vi "Columns.vi"() -> (2 "Columns":T1)   [LabVIEW 2020, in "Test.lvlib" / "Player.lvclass"]
uses:
  Player.lvclass
  Player.lvclass/Player.ctl
  <vilib>/IlluminatedG/IG Conditum Base/Conditum/Columns/Type/Definition.ctl
  <vilib>/IlluminatedG/IG Conditum Base/Conditum/Columns/Type/Type.lvclass
  <vilib>/IlluminatedG/IG Conditum Base/Conditum/Attributes.ctl
  <vilib>/IlluminatedG/IG Conditum Base/Conditum/Conditum.lvlib
  <vilib>/IlluminatedG/IG Conditum Base/Conditum/Columns/String/Definition.ctl
  <vilib>/IlluminatedG/IG Conditum Base/Conditum/Columns/String/String.lvclass
  <vilib>/IlluminatedG/IG Conditum Base/Conditum/Columns/String/String Definition.ctl
  <vilib>/IlluminatedG/IG Conditum Base/Conditum/Columns/Double/Definition.ctl
  <vilib>/IlluminatedG/IG Conditum Base/Conditum/Columns/Double/Double.lvclass
  <vilib>/IlluminatedG/IG Conditum Base/Conditum/Columns/Double/Double Definition.ctl
  <vilib>/IlluminatedG/IG Conditum Base/Conditum/Columns/Boolean/Definition.ctl
  <vilib>/IlluminatedG/IG Conditum Base/Conditum/Columns/Boolean/Boolean.lvclass
  <vilib>/IlluminatedG/IG Conditum Base/Conditum/Columns/Boolean/Boolean Definition.ctl
  C:/Program Files (x86)/National Instruments/LabVIEW 2020/vi.lib/IlluminatedG/IG Conditum Base/Conditum/Columns/Type/Type.lvclass
  C:/Program Files (x86)/National Instruments/LabVIEW 2020/vi.lib/IlluminatedG/IG Conditum Base/Conditum/Columns/String/String.lvclass
  C:/Program Files (x86)/National Instruments/LabVIEW 2020/vi.lib/IlluminatedG/IG Conditum Base/Conditum/Columns/Double/Double.lvclass
  C:/Program Files (x86)/National Instruments/LabVIEW 2020/vi.lib/IlluminatedG/IG Conditum Base/Conditum/Columns/Boolean/Boolean.lvclass
  Columns.ctl
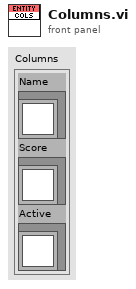
[diagram p1: front panel]
types:
  T1 = typedef "Test.lvlib/Player.lvclass/Columns.ctl" = cluster{"Name":refnum<class "String.lvclass">, "Score":refnum<class "Double.lvclass">, "Active":refnum<class "Boolean.lvclass">}
  T2 = typedef "Conditum.lvlib/Columns.lvlib/Boolean.lvclass/Boolean Definition.ctl" = cluster{"Type":T3, "Attributes":T4, "Boolean":T5}
  T3 = typedef "Conditum.lvlib/Columns.lvlib/Type.lvclass/Definition.ctl" = cluster{"Name":string, "Nullable":bool, "Default NULL":bool}
  T4 = typedef "Conditum.lvlib/Attributes.ctl" = cluster{"Primary Key":bool, "Unique":bool, "Foreign Key":bool, "Auto Increment":bool}
  T5 = typedef "Conditum.lvlib/Columns.lvlib/Boolean.lvclass/Definition.ctl" = cluster{"Default":bool}
  T6 = typedef "Conditum.lvlib/Columns.lvlib/Double.lvclass/Double Definition.ctl" = cluster{"Type":T3, "Attributes":T4, "Double":T7}
  T7 = typedef "Conditum.lvlib/Columns.lvlib/Double.lvclass/Definition.ctl" = cluster{"Default":dbl}
  T8 = typedef "Conditum.lvlib/Columns.lvlib/String.lvclass/String Definition.ctl" = cluster{"Type":T3, "Attributes":T4, "String":T9}
  T9 = typedef "Conditum.lvlib/Columns.lvlib/String.lvclass/Definition.ctl" = cluster{"Default":string, "Length":i32}
  T10 = cluster{"String out":refnum<class "String.lvclass">, "Double out":refnum<class "Double.lvclass">, "Boolean out":refnum<class "Boolean.lvclass">}
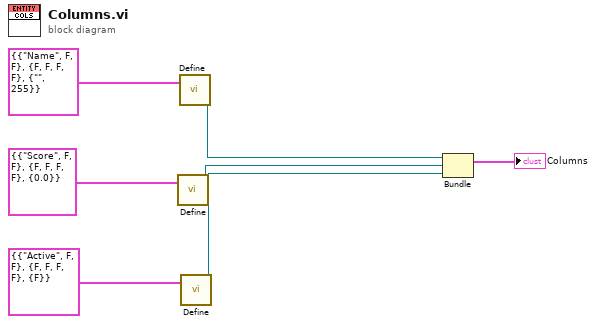
[diagram p0: block diagram]
diagram:
  n1 = call <vilib>:"Define.vi"("Double Definition"=T6 {"Type"={"Name"="Score", "Nullable"=FALSE, "Default NULL"=FALSE}, "Attributes"={"Primary Key"=FALSE, "Unique"=FALSE, "Foreign Key"=FALSE, "Auto Increment"=FALSE}, "Double"={"Default"=0.0}}) -> ("Double out"=w3:refnum<class "Double.lvclass">)  [unwired: 10 in]
  n2 = call <vilib>:"Define.vi"("Definition"=T8 {"Type"={"Name"="Name", "Nullable"=FALSE, "Default NULL"=FALSE}, "Attributes"={"Primary Key"=FALSE, "Unique"=FALSE, "Foreign Key"=FALSE, "Auto Increment"=FALSE}, "String"={"Default"="", "Length"=255}}) -> ("String out"=w5:refnum<class "String.lvclass">)  [unwired: 10 in]
  n3 = call <vilib>:"Define.vi"("Init Data"=T2 {"Type"={"Name"="Active", "Nullable"=FALSE, "Default NULL"=FALSE}, "Attributes"={"Primary Key"=FALSE, "Unique"=FALSE, "Foreign Key"=FALSE, "Auto Increment"=FALSE}, "Boolean"={"Default"=FALSE}} ("Definition")) -> ("Boolean out"=w1:refnum<class "Boolean.lvclass">)  [unwired: 10 in]
  n4 = Bundle("String out"=w5, "Double out"=w3, "Boolean out"=w1) -> (→"Columns":T10)  [unwired: 1 in]
